vi "Release.vi"(8 "error in (no error)":errorcluster, 11 "Instrument":refnum<k24>) -> (0 "error out":errorcluster)   [LabVIEW 2011]
doc: "Releases an instrument, always needed in combination with Connect subVI."
uses:
  C:/Program Files/Metrohm Autolab/Autolab SDK 1.10/EcoChemie.Autolab.Sdk.dll
  EcoChemie.Autolab.Sdk.dll
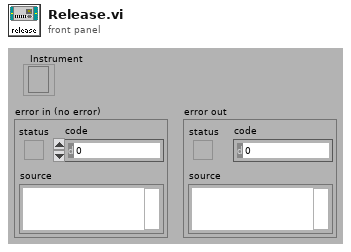
[diagram p1: front panel]
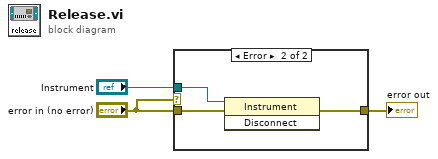
[diagram p0: block diagram]
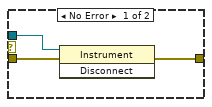
[diagram p2: hidden frame]
diagram:
  n1 = case shown="Error" "error in (no error)" {
    tunnel: "Instrument" -> [w6 w8]
    tunnel: "error in (no error)" -> [w5 w9]
    tunnel: [w4 w7] -> w1
    frame No Error {
      n2 = invoke class="Instrument" method="Disconnect"(reference=w6, error in=w5) -> (error out=w4:errorcluster)  [unwired: 1 in, 2 out]
    }
    frame Error {
      n3 = invoke class="Instrument" method="Disconnect"(reference=w8, error in=w9) -> (error out=w7:errorcluster)  [unwired: 1 in, 2 out]
    }
  }
  "error out" <- w1
